vi "move lorentzian.vi"(7 "action":T1(ring)=enum."replace z(inf)  -- keeping z(center) the same", 8 "new z(center)":cdb, 9 "new z(inf)":cdb, 11 "lorentzian in":T2={"Amplitude"=-1.0311345636926572, "omega(0)"=-1.0311345636926572, "Gamma"=-1.0311345636926572, "phase"=-1.0311345636926572, "Q"=-1.0311345636926572, "Norm  Ampl"=-1.0311345636926572, "z (inf)"=-1.0311345636926572+0.0i, "4corners"={"z (-pi/2)"=-1.0311345636926572+0.5736824521422934i, "z(inf)"=-0.5200164984937075+1.0975277942502903i, "z (pi/2)"=-1.0311345636926572+0.5736824521422934i, "z center"=-0.5136528600391839+0.580046090596817i, "z(0)"=-0.5200164984937075+1.0975277942502903i, "radius"=-1.0311345636926572}} {"z (inf)" format="%#9_9f"; "Q" format="%#9_9f"; "phase" format="%#9_9f"; "Gamma" format="%#9_9f"; "omega(0)" format="%#9_9f"}) -> (3 "lorentzian out":T2={"Amplitude"=-1.0311345636926572, "omega(0)"=-1.0311345636926572, "Gamma"=-1.0311345636926572, "phase"=-1.0311345636926572, "Q"=-1.0311345636926572, "Norm  Ampl"=-1.0311345636926572, "z (inf)"=-1.0311345636926572+0.0i, "4corners"={"z (-pi/2)"=-1.0311345636926572+0.5736824521422934i, "z(inf)"=-0.5200164984937075+1.0975277942502903i, "z (pi/2)"=-1.0311345636926572+0.5736824521422934i, "z center"=-0.5136528600391839+0.580046090596817i, "z(0)"=-0.5200164984937075+1.0975277942502903i, "radius"=-1.0311345636926572}} {"z (inf)" format="%#9_9f"; "Q" format="%#9_9f"; "phase" format="%#9_9f"; "Gamma" format="%#9_9f"; "omega(0)" format="%#9_9f"})   [LabVIEW 2015]
uses:
  lorentzian.ctl
  circle corners.ctl
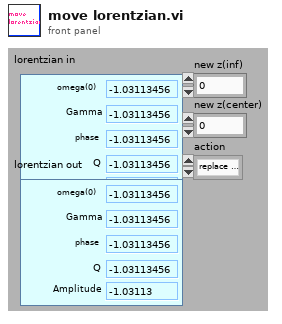
[diagram p1: front panel]
types:
  T1 = enum16{"replace z(center) -- keepin z(inf) the same", "replace z(inf)  -- keeping z(center) the same"}
  T2 = typedef "lorentzian.ctl" = cluster{"Amplitude":dbl, "omega(0)":dbl, "Gamma":dbl, "phase":dbl, "Q":dbl, "Norm  Ampl":dbl, "z (inf)":cdb, "4corners":T3}
  T3 = typedef "circle corners.ctl" = cluster{"z (-pi/2)":cdb, "z(inf)":cdb, "z (pi/2)":cdb, "z center":cdb, "z(0)":cdb, "radius":dbl}
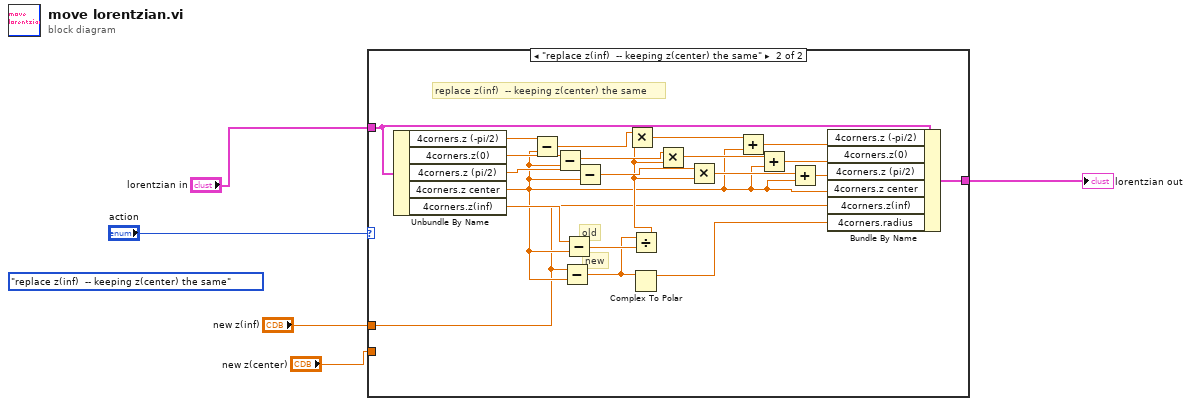
[diagram p0: block diagram]
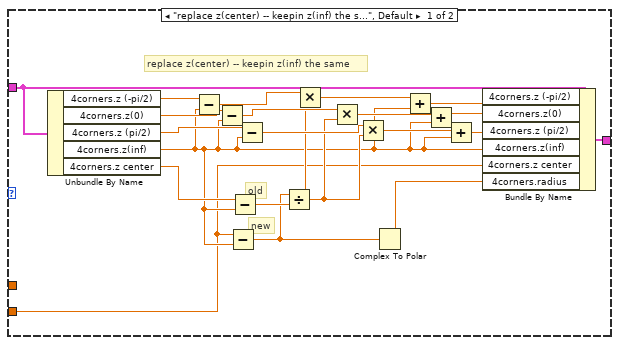
[diagram p2: hidden frame]
diagram:
  (unwired) T1."replace z(inf)  -- keeping z(center) the same" ("Enum")
  n1 = case shown="\"replace z(inf)  -- keeping z(center) the same\"" "action" {
    tunnel: "lorentzian in" -> [w13 w34]
    tunnel: [w6 w28] -> w4
    tunnel: "new z(inf)" -> [_ w27]
    tunnel: "new z(center)" -> [w7 _]
    frame "replace z(center) -- keepin z(inf) the same", Default {
      # "new"
      # "old"
      # "replace z(center) -- keepin z(inf) the same"
      n2 = Unbundle By Name(w13) -> ("4corners.z (-pi/2)"=w11:cdb, "4corners.z(0)"=w10:cdb, "4corners.z (pi/2)"=w9:cdb, "4corners.z(inf)"=w8:cdb, "4corners.z center"=w12:cdb)
      n3 = Subtract(x=w11, y=w8) -> (x-y=w22:cdb)
      n4 = Subtract(x=w10, y=w8) -> (x-y=w21:cdb)
      n5 = Subtract(x=w7, y=w8) -> (x-y=w15:cdb)
      n6 = Subtract(x=w12, y=w8) -> (x-y=w23:cdb)
      n7 = Subtract(x=w9, y=w8) -> (x-y=w20:cdb)
      n8 = Divide(x=w15, y=w23) -> (x/y=w19:cdb)
      n9 = Multiply(x=w22, y=w19) -> (x*y=w18:cdb)
      n10 = Multiply(x=w21, y=w19) -> (x*y=w17:cdb)
      n11 = Multiply(x=w20, y=w19) -> (x*y=w16:cdb)
      n12 = Complex To Polar(r * e^(i*theta)=w15) -> (r=w14:dbl)  [unwired: 1 out]
      n13 = Add(x=w18, y=w8) -> (x+y=w24:cdb)
      n14 = Add(x=w17, y=w8) -> (x+y=w25:cdb)
      n15 = Add(x=w16, y=w8) -> (x+y=w26:cdb)
      n16 = Bundle By Name(cluster=w13, "4corners.z (-pi/2)"=w24, "4corners.z(0)"=w25, "4corners.z (pi/2)"=w26, "4corners.z(inf)"=w8, "4corners.z center"=w7, "4corners.radius"=w14) -> (w6:T2)
    }
    frame "replace z(inf)  -- keeping z(center) the same" {
      # "new"
      # "old"
      # "replace z(inf)  -- keeping z(center) the same"
      n17 = Unbundle By Name(w34) -> ("4corners.z (-pi/2)"=w32:cdb, "4corners.z(0)"=w31:cdb, "4corners.z (pi/2)"=w30:cdb, "4corners.z center"=w29:cdb, "4corners.z(inf)"=w33:cdb)
      n18 = Subtract(x=w32, y=w29) -> (x-y=w44:cdb)
      n19 = Subtract(x=w31, y=w29) -> (x-y=w43:cdb)
      n20 = Subtract(x=w27, y=w29) -> (x-y=w37:cdb)
      n21 = Subtract(x=w33, y=w29) -> (x-y=w45:cdb)
      n22 = Subtract(x=w30, y=w29) -> (x-y=w42:cdb)
      n23 = Divide(x=w37, y=w45) -> (x/y=w41:cdb)
      n24 = Multiply(x=w44, y=w41) -> (x*y=w40:cdb)
      n25 = Complex To Polar(r * e^(i*theta)=w37) -> (r=w36:dbl)  [unwired: 1 out]
      n26 = Multiply(x=w43, y=w41) -> (x*y=w39:cdb)
      n27 = Multiply(x=w42, y=w41) -> (x*y=w38:cdb)
      n28 = Add(x=w40, y=w29) -> (x+y=w46:cdb)
      n29 = Add(x=w39, y=w29) -> (x+y=w35:cdb)
      n30 = Add(x=w38, y=w29) -> (x+y=w47:cdb)
      n31 = Bundle By Name(cluster=w34, "4corners.z (-pi/2)"=w46, "4corners.z(0)"=w35, "4corners.z (pi/2)"=w47, "4corners.z center"=w29, "4corners.z(inf)"=w27, "4corners.radius"=w36) -> (w28:T2)
    }
  }
  "lorentzian out" <- w4
